vi "Send RX Message.vi"(8 "error in (no error)":errorcluster, 11 "RxTx in":refnum<class "CM_RxTx.lvclass">) -> (0 "error out":errorcluster, 3 "RxTx out":refnum<class "CM_RxTx.lvclass">)   [LabVIEW 2018, in "CM_RxTx.lvclass"]
doc: "Send Rx Message"
uses:
  CM_RxTx.lvclass
  CM_RxTx.lvclass/CM_RxTx.ctl
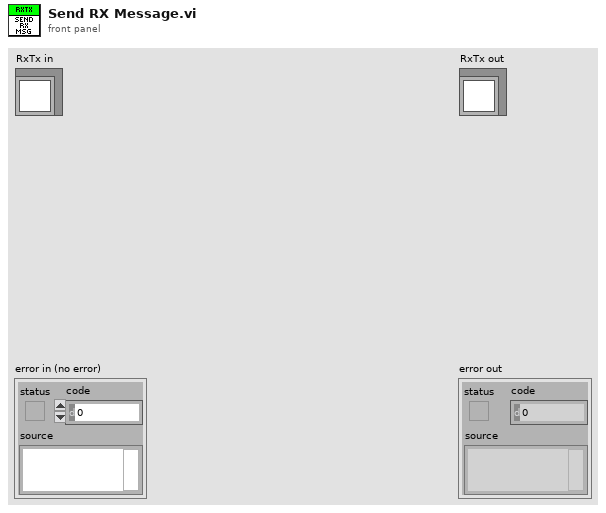
[diagram p1: front panel]
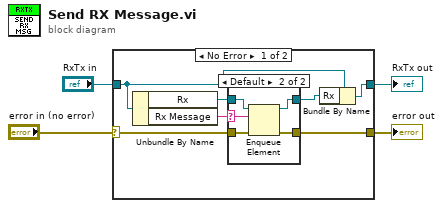
[diagram p0: block diagram]
diagram:
  n1 = case shown="No Error" "error in (no error)" {
    selector: "error in (no error)" -> [w10 w20]
    tunnel: [w11 w20] -> w2
    tunnel: [w5 w19] -> w1
    tunnel: "RxTx in" -> [w7 w19]
    frame No Error {
      n2 = Unbundle By Name(w7) -> ("Rx"=w9:refnum<queue>, "Rx Message"=w8:string)
      n3 = case shown="Default" w8 {
        selector: w8 -> [_ w14]
        tunnel: [w13 w18] -> w11
        tunnel: w10 -> [w13 w17]
        tunnel: w9 -> [w12 w16]
        tunnel: [w12 w15] -> w6
        frame "" {
        }
        frame Default {
          n4 = Enqueue Element(queue=w16, element=w14, error in (no error)=w17) -> (queue out=w15:refnum<queue>, error out=w18:errorcluster)  [unwired: 1 in, 1 out]
        }
      }
      n5 = Bundle By Name(cluster=w7, "Rx"=w6) -> (w5:refnum<class "CM_RxTx.lvclass">)
    }
    frame Error {
    }
  }
  "error out" <- w2
  "RxTx out" <- w1
